vi "color trip.vi"() -> ()   [LabVIEW 2022 SP3]
panel:
  out "Color Box":u32(colorbox)
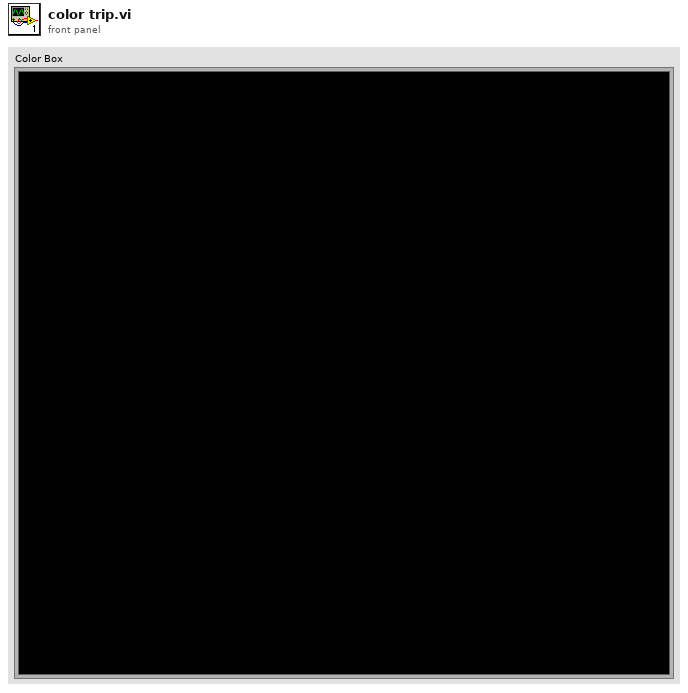
[diagram p1: front panel]
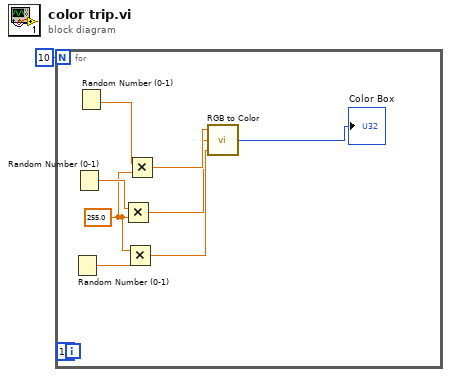
[diagram p0: block diagram]
diagram:
  n1 = for {
    N: 10 -> [_]
    (unwired) 10
    w5 = 255.0 ("y")
    n2 = Random Number (0-1)() -> (number: 0 to 1=w6:dbl)
    n3 = Random Number (0-1)() -> (number: 0 to 1=w7:dbl)
    n4 = Random Number (0-1)() -> (number: 0 to 1=w8:dbl)
    n5 = Multiply(x=w7, y=w5) -> (x*y=w3:dbl)
    n6 = Multiply(x=w5, y=w6) -> (x*y=w2:dbl)
    n7 = Multiply(x=w8, y=w5) -> (x*y=w4:dbl)
    n8 = call <vilib>:"RGB to Color.vi"("B"=w2, "G"=w3, "R"=w4) -> ("Color"=→"Color Box":u32)
  }
